vi "GetControlFromTabControl.vi"(2 "error in":errorcluster, 4 "Control Name":string, 5 "Ctl Refnum":refnum<vi>) -> (0 "error out":errorcluster, 1 "CtlRef":refnum<vi>)   [LabVIEW 2018]
panel:
  out "Array":string[](array[string])
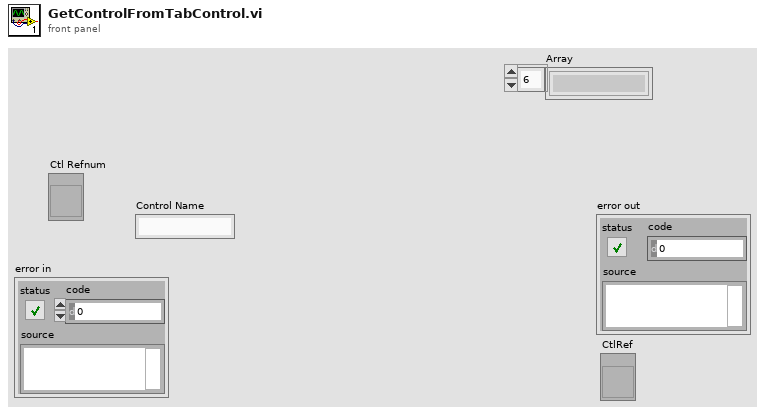
[diagram p1: front panel]
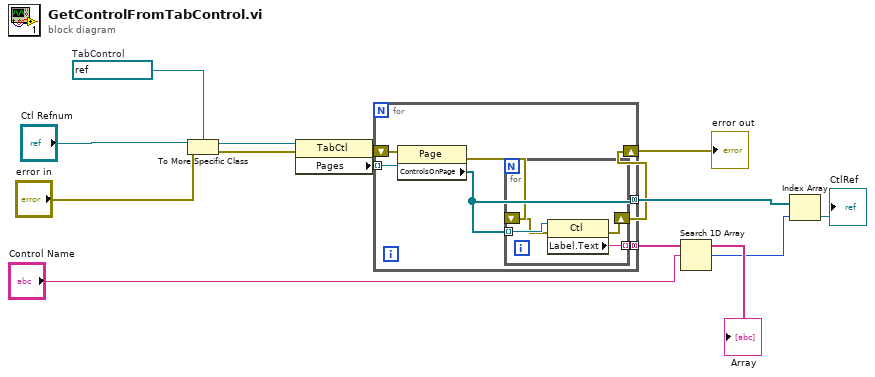
[diagram p0: block diagram]
diagram:
  w13 = refnum<vi> refnum  # TabControl
  n1 = To More Specific Class(target class=w13, reference="Ctl Refnum", error in="error in") -> (specific class reference=w12:refnum<vi>, error out=w11:errorcluster)
  n2 = property class="TabCtl"(reference=w12, error in=w11) -> (error out=w2:errorcluster, "Pages"=w4:refnum<vi>[])  [unwired: 1 out]
  n3 = for {
    tunnel: [w19] -> w9 mode=concatenating
    tunnel: [w18] -> w7 mode=concatenating
    tunnel: w4 -> [w17] mode=indexing
    shift-right: [w16] -> w3
    shift-left: w2 -> [w15]
    n4 = property class="Page"(reference=w17, error in=w15) -> (error out=w14:errorcluster, "ControlsOnPage"=w18:refnum<vi>[])  [unwired: 1 out]
    n5 = for {
      tunnel: w18 -> [w23] mode=indexing
      tunnel: [w22] -> w19 mode=indexing
      shift-right: [w21] -> w16
      shift-left: w14 -> [w20]
      n6 = property class="Ctl"(reference=w23, error in=w20) -> (error out=w21:errorcluster, "Label.Text"=w22:string)  [unwired: 1 out]
    }
  }
  "error out" <- w3
  "Array" <- w9
  n7 = Search 1D Array(1D array=w9, element="Control Name") -> (index of element=w6:i32)  [unwired: 1 in]
  n8 = Index Array(array=w7, index=w6) -> (element=→"CtlRef":refnum<vi>)
